vi "Task Type.vi"(11 "DaqAnalogIn in":refnum<class "DaqAnalogIn.lvclass">) -> (2 "Task Type":string)   [LabVIEW 2020, in "VolatusDaq.lvlib" / "DaqAnalogIn.lvclass"]
uses:
  DaqAnalogIn.lvclass
  DaqAnalogIn.lvclass/DaqAnalogIn.ctl
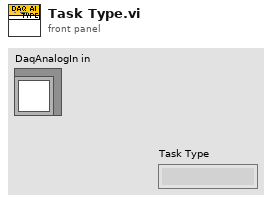
[diagram p1: front panel]
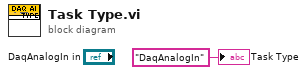
[diagram p0: block diagram]
diagram:
  "Task Type" <- "DaqAnalogIn" ("Task Type")
